vi "AddConnection.vi"(8 "error in (no error)":errorcluster, 10 "Connection":T1={"Connection Handlers's Enqueuer"=refnum, "Connection Window's Enqueuer"=refnum, "Connection Information"={"Connection number"=-1, "Remote Address"="", "Remote Port"=0, "Connection ID"=refnum}}, 11 "TCP_Server in":refnum<class "TCP_Server.lvclass">) -> (0 "error out":errorcluster, 3 "TCP_Server out":refnum<class "TCP_Server.lvclass">)   [LabVIEW 2023, in "TCP_Server.lvlib" / "TCP_Server.lvclass"]
uses:
  TCP_Server.lvclass
  C:/Program Files (x86)/National Instruments/LabVIEW 2023/vi.lib/ActorFramework/Actor/Actor.lvclass
  TypeDeclarations/ServerConnection.ctl
  <vilib>/ActorFramework/Message Enqueuer/Message Enqueuer.lvclass
  TCP_Listener/TypeDefinitions/ConnectionInformation.ctl
  <vilib>/ActorFramework/Actor/Actor.lvclass/Actor.ctl
  <vilib>/ActorFramework/Message Enqueuer/Message Enqueuer.lvclass/Message Enqueuer.ctl
  TCP_Server.lvclass/TCP_Server.ctl
  TCP_serverGUI/TCP_serverGUI Messages/UpdateConnectionsListbox Msg/UpdateConnectionsListbox Msg.lvclass/UpdateConnectionsListbox Msg.ctl
  <vilib>/ActorFramework/Message Enqueuer/Init from Existing Queue.vi
  <vilib>/ActorFramework/Message Enqueuer/Enqueue.vi
  TCP_Server Messages/AddConnectionHandler Msg/AddConnectionHandler Msg.lvclass
  C:/Program Files (x86)/National Instruments/LabVIEW 2023/vi.lib/ActorFramework/Message/Message.lvclass
  TCP_serverGUI/TCP_serverGUI Messages/UpdateConnectionsListbox Msg/UpdateConnectionsListbox Msg.lvclass
  <vilib>/ActorFramework/Message Priority Queue/Priority Enqueue.vi
  <vilib>/ActorFramework/Actor/Actor.lvclass
  TCP_Server Messages/UpdateGUIconnectionTable Msg/UpdateGUIconnectionTable Msg.lvclass
  TCP_Server.lvlib
  TCP_Listener/TCP_Listener.lvlib
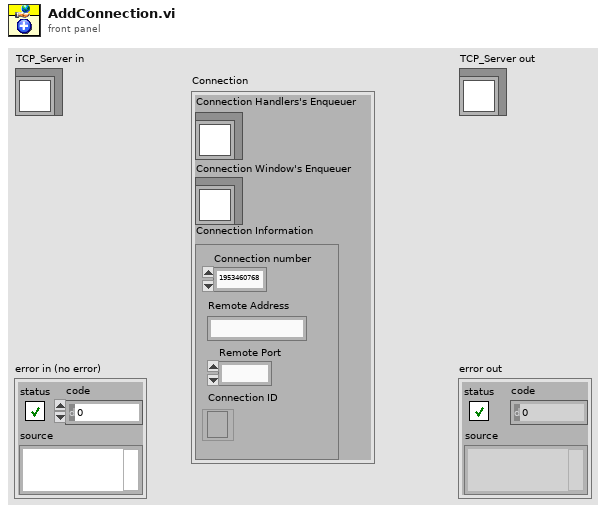
[diagram p1: front panel]
types:
  T1 = typedef "TCP_Server.lvlib/ServerConnection.ctl" = cluster{"Connection Handlers's Enqueuer":refnum<class "Message Enqueuer.lvclass">, "Connection Window's Enqueuer":refnum<class "Message Enqueuer.lvclass">, "Connection Information":T2}
  T2 = typedef "TCP_Listener.lvlib/ConnectionInformation.ctl" = cluster{"Connection number":i32, "Remote Address":string, "Remote Port":u16, "Connection ID":refnum<k5>}
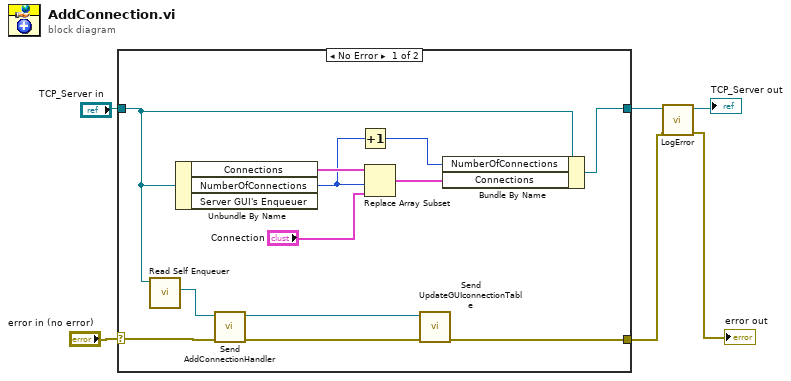
[diagram p0: block diagram]
diagram:
  n1 = case shown="No Error" "error in (no error)" {
    selector: "error in (no error)" -> [w15 w20]
    tunnel: [w7 w20] -> w2
    tunnel: [w18 w19] -> w4
    tunnel: "TCP_Server in" -> [w17 w19]
    frame No Error {
      n2 = call <vilib>:"Read Self Enqueuer.vi"("Actor"=w17) -> ("Self Enqueuer"=w16:refnum<class "Message Enqueuer.lvclass">)  [unwired: 10 in]
      n3 = Unbundle By Name(w17) -> ("Connections"=w12:T1[], "NumberOfConnections"=w11:i32)  [unwired: 1 out]
      n4 = call "Send AddConnectionHandler.vi"("error in (no error)"=w15, "Message Enqueuer"=w16) -> ("error out"=w8:errorcluster, "Message Enqueuer out"=w9:refnum<class "Message Enqueuer.lvclass">)  [unwired: 8 in]
      n5 = Increment(x=w11) -> (x+1=w14:i32)
      n6 = Replace Array Subset(array=w12, new element="Connection", index=w11) -> (w10:T1[])
      n7 = call "Send UpdateGUIconnectionTable.vi"("error in (no error)"=w8, "Message Enqueuer"=w9) -> ("error out"=w7:errorcluster)  [unwired: 8 in, 1 out]
      n8 = Bundle By Name(cluster=w17, "NumberOfConnections"=w14, "Connections"=w10) -> (w18:refnum<class "TCP_Server.lvclass">)
    }
    frame Error {
    }
  }
  n9 = call "LogError.vi"("error in (no error)"=w2, "TCP_Server in"=w4) -> ("error out"=→"error out":errorcluster, "TCP_Server out"=→"TCP_Server out":refnum<class "TCP_Server.lvclass">)  [unwired: 8 in]
